vi "losowe3_PH.vi"() -> ()   [LabVIEW 2021]
uses:
  <vilib>/Analysis/baseanly.llb/Mean (DBL).vi
  <vilib>/Utility/file.llb/Write Delimited Spreadsheet (DBL).vi
  <vilib>/Analysis/NI_AALBase.lvlib
panel:
  out "Wartoœæ œrednia":dbl format="%0.2f"
  out "Liczby losowe":dbl(graph)
  in  "stop":bool
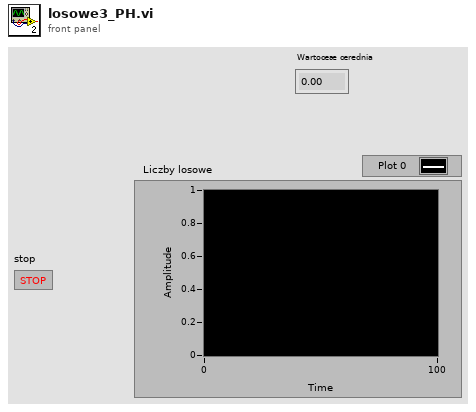
[diagram p1: front panel]
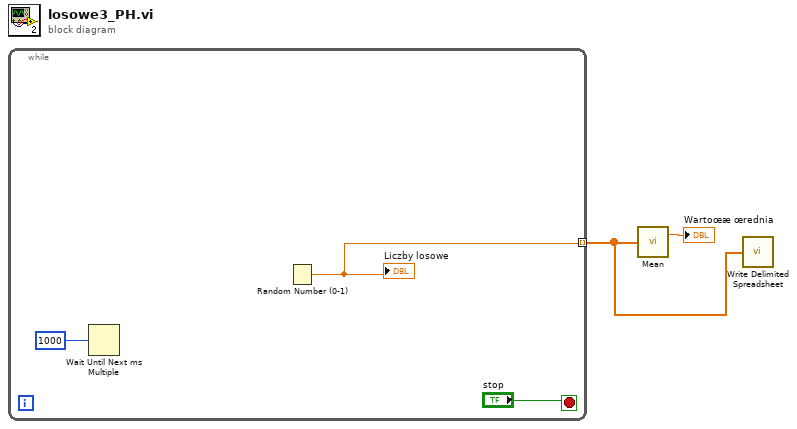
[diagram p0: block diagram]
diagram:
  n1 = while {
    tunnel: [w3] -> w1 mode=indexing
    stop <- "stop" stop-if-true
    n2 = Wait Until Next ms Multiple(millisecond multiple=u32 1000 ("millisecond timer value")) -> ()  [unwired: 1 out]
    n3 = Random Number (0-1)() -> (number: 0 to 1=w3:dbl)
    "Liczby losowe" <- w3
  }
  n4 = call-poly <vilib>:"Mean.vi"("X"=w1) -> ("mean"=→"Wartoœæ œrednia":dbl)  [unwired: 1 out]
  n5 = call-poly <vilib>:"Write Delimited Spreadsheet.vi"("1D data"=w1) -> ()  [unwired: 13 in, 2 out]
